vi "Chapter 22 - Nutation and the Obliquity of the Ecliptic.vi"(0 "T":dbl=-0.12729637234770705 format="%#_12g") -> (4 "series sum for d(psi) [\"]":dbl=-3.7689843372488014 format="%#_4g", 6 "series sum for d(epsilon) [\"]":dbl=9.447598043682703 format="%#_4g", 8 "Laskar True Obliquity [DMS]":string="23:26:36.854", 10 "Laskar True Obliquity [Deg]":dbl=23.44357062374612 format="%#_10g")   [LabVIEW 2015]
panel:
  out "epsilon-not":string="23:26:27.407"
  out "Series of Coeffs\nShowing Convergence":dbl[](array[numeric])=[-33568.15989554565, -7638.602762626091, 1759.1796746931293, 789.3080064806869, 1420.1874876506618, -539.626324854248, -393.73600076284373, 340.6445472084611, 228.12446606661692, -187.07577516388326, 111.03088136782891, 52.77081108289655, 121.14755950731983, -62.85226224030107, -54.860536706122645, 6.1997544482272255, -35.736408899524854, -11.171072114280271, -3.876438130288009, -15.364250599505915, 26.035312746981635, -22.993561341985, 28.677194650167454, -28.874880781724638, -24.88823194212684, -4.908204937014608, 19.577538254599077]
  in  "Arguments of Parameter Multiples":dbl[][](array[numeric])=[[0.0, 0.0, 0.0, 0.0, 1.0, -171996.0, -174.2, 92025.0, 8.9], [-2.0, 0.0, 0.0, 2.0, 2.0, -13187.0, -1.6, 5736.0, -3.1], [0.0, 0.0, 0.0, 2.0, 2.0, -2274.0, -0.2, 977.0, -0.5], [0.0, 0.0, 0.0, 0.0, 2.0, 2062.0, 0.2, -895.0, 0.5], [0.0, 1.0, 0.0, 0.0, 0.0, 1426.0, -3.4, 54.0, -0.1], [0.0, 0.0, 1.0, 0.0, 0.0, 712.0, 0.1, -7.0, 0.0], [-2.0, 1.0, 0.0, 2.0, 2.0, -517.0, 1.2, 224.0, -0.6], [0.0, 0.0, 0.0, 2.0, 1.0, -386.0, -0.4, 200.0, 0.0], [0.0, 0.0, 1.0, 0.0, 0.0, -301.0, 0.0, 129.0, -0.1], [-2.0, -1.0, 0.0, 2.0, 2.0, 217.0, -0.5, -95.0, 0.3], [-2.0, 0.0, 1.0, 0.0, 0.0, -158.0, 0.0, 0.0, 0.0], [-2.0, 0.0, 0.0, 2.0, 1.0, 129.0, 0.1, -70.0, 0.0], [0.0, 0.0, -1.0, 2.0, 2.0, 123.0, 0.0, -53.0, 0.0], [2.0, 0.0, 0.0, 0.0, 0.0, 63.0, 0.0, 0.0, 0.0], [0.0, 0.0, 1.0, 0.0, 1.0, 63.0, 0.1, -33.0, 0.0], [2.0, 0.0, -1.0, 2.0, 2.0, -59.0, 0.0, 26.0, 0.0], [0.0, 0.0, -1.0, 0.0, 1.0, -58.0, -0.1, 32.0, 0.0], [0.0, 0.0, 1.0, 2.0, 1.0, -51.0, 0.0, 27.0, 0.0], [-2.0, 0.0, 2.0, 0.0, 0.0, 48.0, 0.0, 0.0, 0.0], [0.0, 0.0, -2.0, 2.0, 1.0, 46.0, 0.0, -24.0, 0.0], [2.0, 0.0, 0.0, 2.0, 2.0, -38.0, 0.0, 16.0, 0.0], [0.0, 0.0, 2.0, 2.0, 2.0, -31.0, 0.0, 13.0, 0.0], [0.0, 0.0, 2.0, 0.0, 0.0, 29.0, 0.0, 0.0, 0.0], [-2.0, 0.0, 1.0, 2.0, 2.0, 29.0, 0.0, -12.0, 0.0], [0.0, 0.0, 0.0, 2.0, 0.0, 26.0, 0.0, 0.0, 0.0], [-2.0, 0.0, 0.0, 2.0, 0.0, -22.0, 0.0, 0.0, 0.0], [0.0, 0.0, -1.0, 2.0, 1.0, 21.0, 0.0, -10.0, 0.0], [0.0, 2.0, 0.0, 0.0, 0.0, 17.0, -0.1, 0.0, 0.0], [2.0, 0.0, -1.0, 0.0, 1.0, 16.0, 0.0, -8.0, 0.0], [-2.0, 2.0, 0.0, 2.0, 2.0, -16.0, 0.1, 7.0, 0.0], [0.0, 1.0, 0.0, 0.0, 1.0, -15.0, 0.0, 9.0, 0.0]]
  out "Laskar Mean Obliquity (epsilon_0)":dbl=23.44094629095621 format="%#_10g"
  out "U":dbl=-0.0012729637234770706
  out "d(epsilon) nutation in obliquity":dbl=9.467983737223694
  out "d(psi)":dbl=-2.3335325915571588
  out "Omega - Longitude of the ascending node of the Moon's mean orbit on the ecliptric":dbl=371.253083202876 format="%#_7g"
  out "F - Moon's argument of latitude":dbl=-61416.5920933594 format="%#_9g"
  out "M' - Mean anomaly of the Moon":dbl=-60610.721587303946 format="%#_9g"
  out "M - Mean anomaly of the Sun (Earth)":dbl=-4225.020798835174 format="%#_8g"
  out "D - Mean elongataion of the Moon from the Sun":dbl=-56383.03768817535 format="%#_9g"
  # "These are all expressed in degrees and calculated according to page 144 in Meeu"
  # "This is 0.005\" different than Meeus.  It could be\nmade better through the addition of more series\nterms but frankly this is probably okay for my work."
  # "Accuracy Can be Increased by adding more series terms from Meeus'\nTable 22.A on pages 145-146"
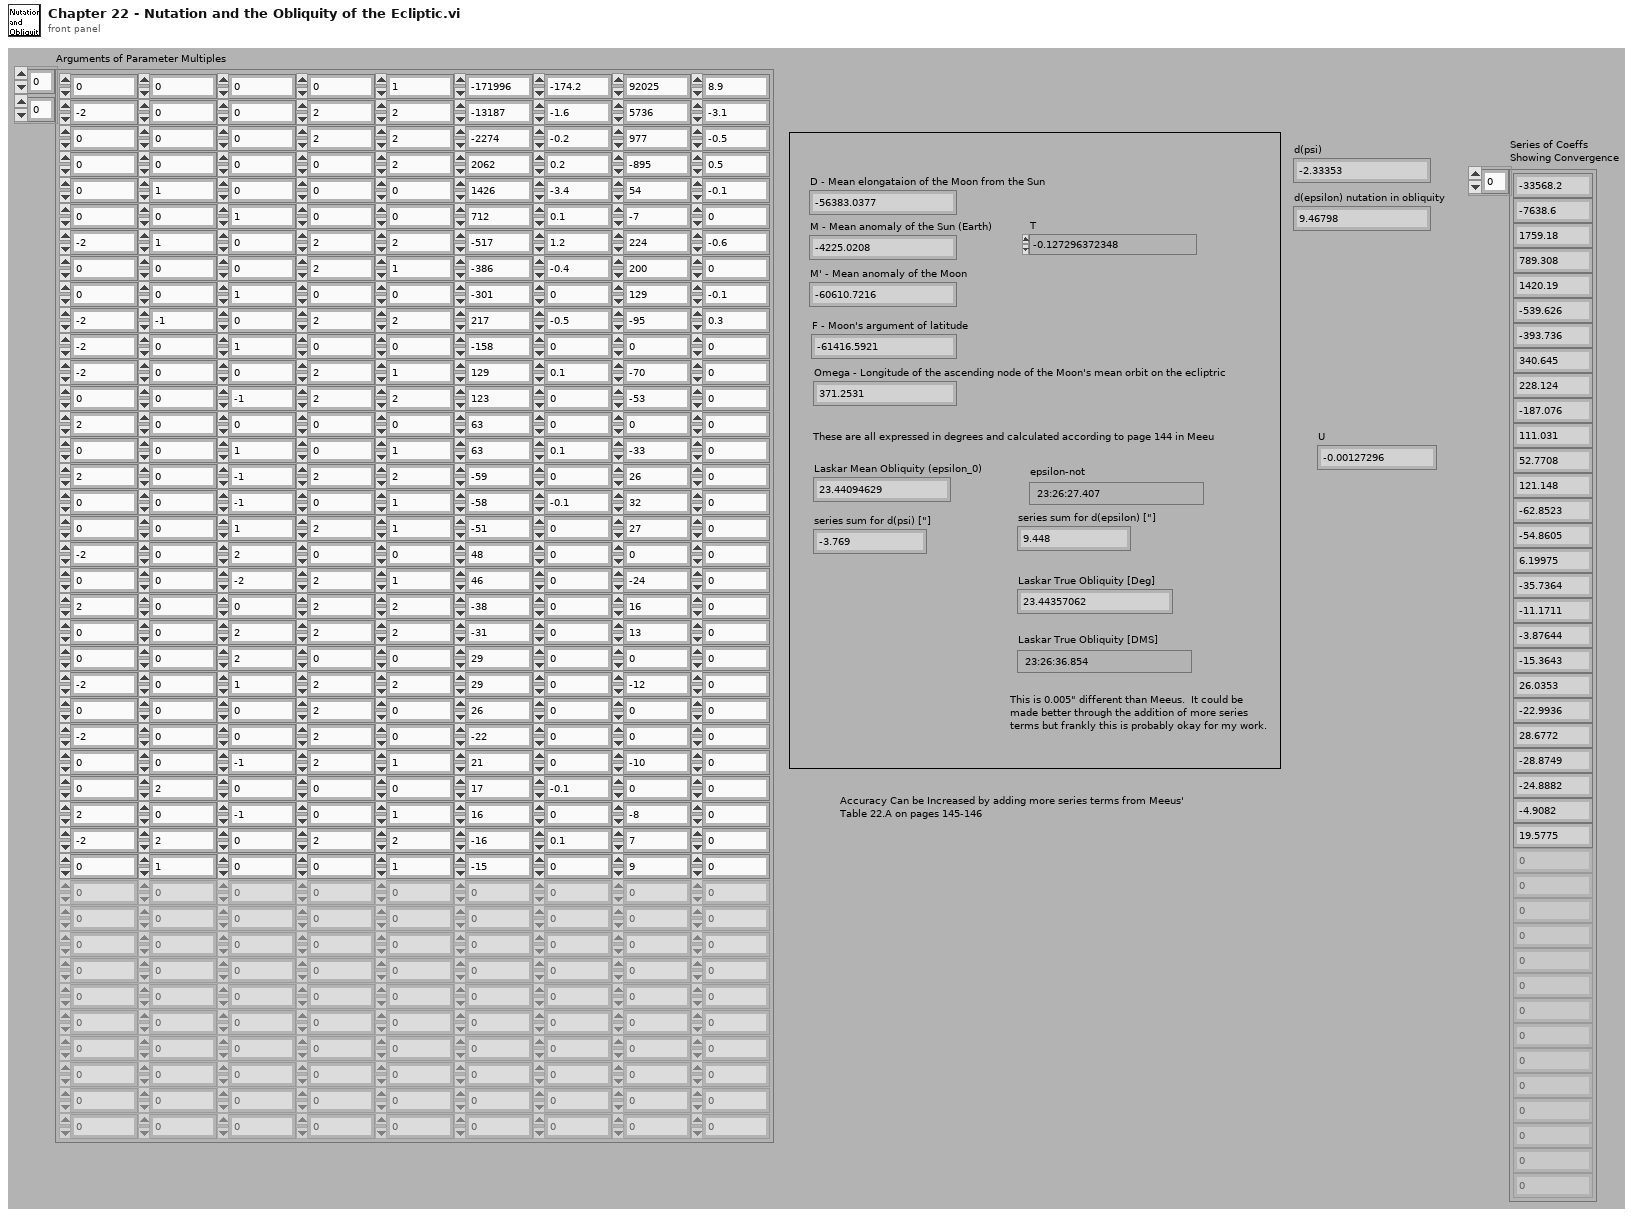
[diagram p1: front panel]
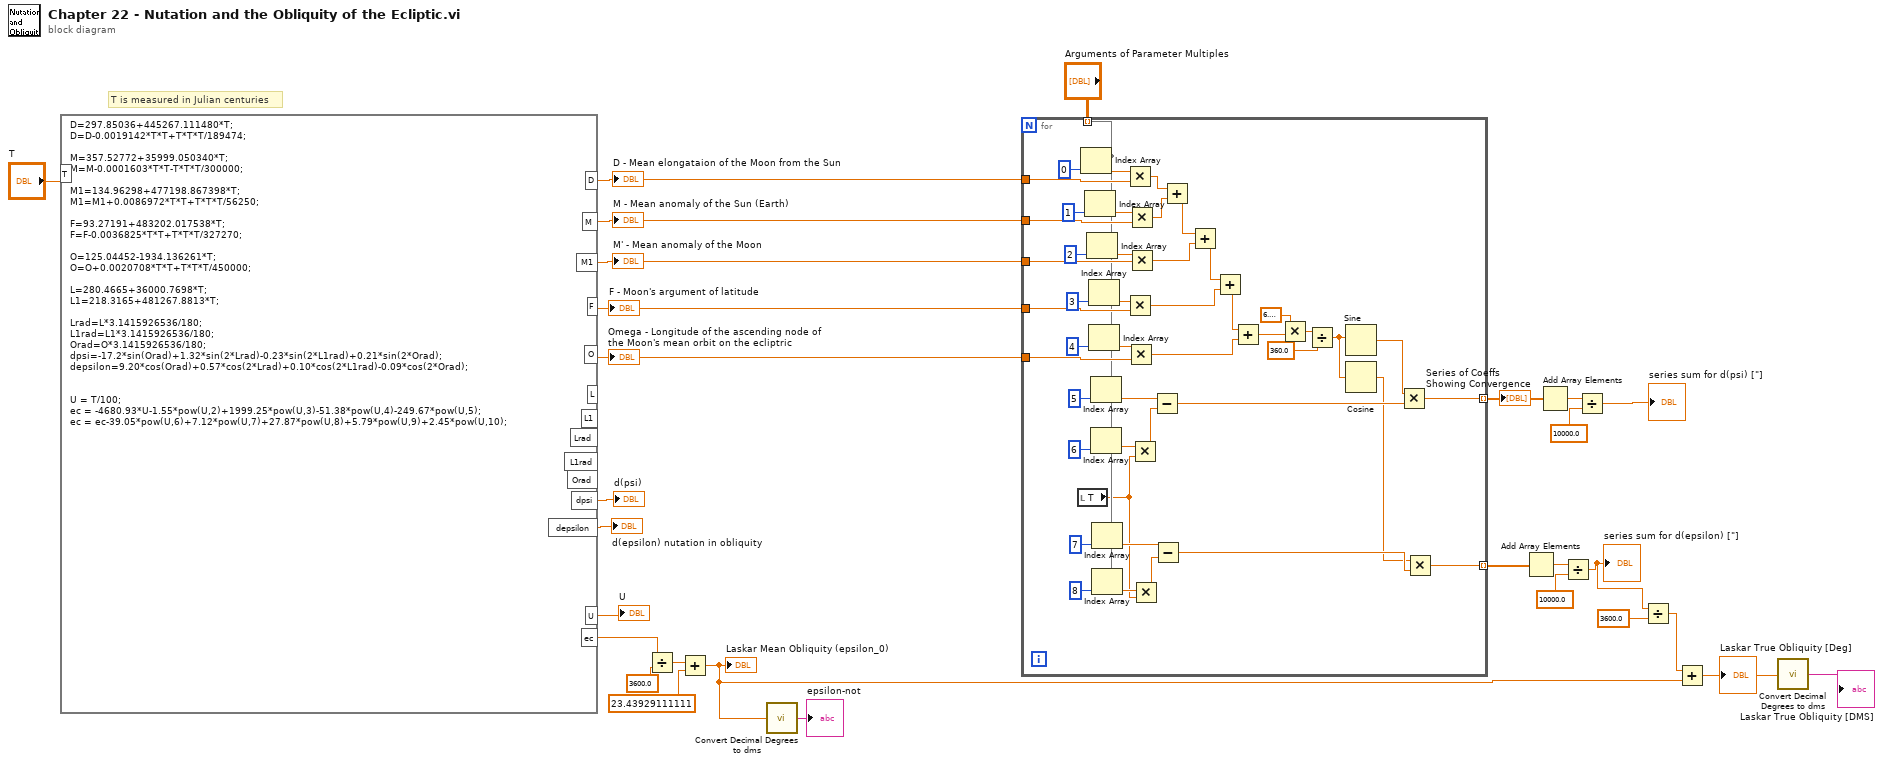
[diagram p0: block diagram]
diagram:
  # "T is measured in Julian centuries"
  n1 = formula code="D=297.85036+445267.111480*T;\nD=D-0.0019142*T*T+T*T*T/189474;\n\nM=357.52772+35999.050340*T;\nM=M-0.0001603*T*T-T*T*T/300000;\n\nM1=134.96298+477198.867398*T;\nM1=M1+0.0086972*T*T+T*T*T/56250;\n\nF=93.27191+483202.017538*T;\nF=F-0.0036825*T*T+T*T*T/327270;\n\nO=125.04452-1934.136261*T;\nO=O+0.0020708*T*T+T*T*T/450000;\n\nL=280.4665+36000.7698*T;\nL1=218.3165+481267.8813*T;\n\nLrad=L*3.1415926536/180;\nL1rad=L1*3.1415926536/180;\nOrad=O*3.1415926536/180;\ndpsi=-17.2*sin(Orad)+1.32*sin(2*Lrad)-0.23*sin(2*L1rad)+0.21*sin(2*Orad);\ndepsilon=9.20*cos(Orad)+0.57*cos(2*Lrad)+0.10*cos(2*L1rad)-0.09*cos(2*Orad);\n\n\nU = T/100;\nec = -4680.93*U-1.55*pow(U,2)+1999.25*pow(U,3)-51.38*pow(U,4)-249.67*pow(U,5);\nec = ec-39.05*pow(U,6)+7.12*pow(U,7)+27.87*pow(U,8)+5.79*pow(U,9)+2.45*pow(U,10);"("T"="T") -> ("D"=w19:dbl, "M"=w18:dbl, "M1"=w17:dbl, "F"=w16:dbl, "O"=w15:dbl, "dpsi"=→"d(psi)":dbl, "depsilon"=→"d(epsilon) nutation in obliquity":dbl, "ec"=w22:dbl, "U"=→"U":dbl)  [unwired: 5 out]
  "D - Mean elongataion of the Moon from the Sun" <- w19
  "M - Mean anomaly of the Sun (Earth)" <- w18
  "M' - Mean anomaly of the Moon" <- w17
  "F - Moon's argument of latitude" <- w16
  "Omega - Longitude of the ascending node of the Moon's mean orbit on the ecliptric" <- w15
  n2 = Divide(x=w22, y=3600.0) -> (x/y=w23:dbl)
  n3 = Add(x=w23, y=23.43929111111) -> (x+y=w2:dbl)
  "Laskar Mean Obliquity (epsilon_0)" <- w2
  n4 = call "Convert Decimal Degrees to dms.vi"("Decimal Degrees"=w2) -> ("Deg:Min:Sec"=→"epsilon-not":string)
  n5 = for {
    tunnel: "Arguments of Parameter Multiples" -> [w35] mode=indexing
    tunnel: w19 -> [w69]
    tunnel: w18 -> [w67]
    tunnel: w17 -> [w64]
    tunnel: w16 -> [w62]
    tunnel: w15 -> [w60]
    tunnel: [w44] -> w14 mode=indexing
    tunnel: [w29] -> w8 mode=indexing
    n6 = local read "T"() -> (w32:dbl)
    n7 = Index Array(array=w35, index=0) -> (element=w68:dbl)
    n8 = Index Array(array=w35, index=1) -> (element=w66:dbl)
    n9 = Index Array(array=w35, index=2) -> (element=w65:dbl)
    n10 = Index Array(array=w35, index=3) -> (element=w63:dbl)
    n11 = Index Array(array=w35, index=4) -> (element=w61:dbl)
    n12 = Index Array(array=w35, index=5) -> (element=w41:dbl)
    n13 = Index Array(array=w35, index=6) -> (element=w42:dbl)
    n14 = Index Array(array=w35, index=7) -> (element=w34:dbl)
    n15 = Index Array(array=w35, index=8) -> (element=w33:dbl)
    n16 = Multiply(x=w68, y=w69) -> (x*y=w59:dbl)
    n17 = Multiply(x=w63, y=w62) -> (x*y=w54:dbl)
    n18 = Multiply(x=w61, y=w60) -> (x*y=w52:dbl)
    n19 = Multiply(x=w66, y=w67) -> (x*y=w58:dbl)
    n20 = Multiply(x=w65, y=w64) -> (x*y=w56:dbl)
    n21 = Multiply(x=w42, y=w32) -> (x*y=w40:dbl)
    n22 = Multiply(x=w33, y=w32) -> (x*y=w38:dbl)
    n23 = Subtract(x=w41, y=w40) -> (x-y=w39:dbl)
    n24 = Subtract(x=w34, y=w38) -> (x-y=w31:dbl)
    n25 = Add(x=w59, y=w58) -> (x+y=w57:dbl)
    n26 = Add(x=w57, y=w56) -> (x+y=w55:dbl)
    n27 = Add(x=w55, y=w54) -> (x+y=w53:dbl)
    n28 = Add(x=w53, y=w52) -> (x+y=w51:dbl)
    n29 = Multiply(x=6.283185307179586, y=w51) -> (x*y=w49:dbl)
    n30 = Divide(x=w49, y=360.0) -> (x/y=w47:dbl)
    n31 = Sine(x=w47) -> (sin(x)=w45:dbl)
    n32 = Cosine(x=w47) -> (cos(x)=w30:dbl)
    n33 = Multiply(x=w45, y=w39) -> (x*y=w44:dbl)
    n34 = Multiply(x=w30, y=w31) -> (x*y=w29:dbl)
  }
  "Series of Coeffs\nShowing Convergence" <- w14
  n35 = Add Array Elements(numeric array=w8) -> (sum=w10:dbl)
  n36 = Add Array Elements(numeric array=w14) -> (sum=w13:dbl)
  n37 = Divide(x=w10, y=10000.0) -> (x/y=w6:dbl)
  "series sum for d(epsilon) [\"]" <- w6
  n38 = Divide(x=w13, y=10000.0) -> (x/y=→"series sum for d(psi) [\"]":dbl)
  n39 = Divide(x=w6, y=3600.0) -> (x/y=w5:dbl)
  n40 = Add(x=w5, y=w2) -> (x+y=w4:dbl)
  "Laskar True Obliquity [Deg]" <- w4
  n41 = call "Convert Decimal Degrees to dms.vi"("Decimal Degrees"=w4) -> ("Deg:Min:Sec"=→"Laskar True Obliquity [DMS]":string)
